vi "Center Front Panel.vi"(8 "error in (no error)":errorcluster, 11 "Actor in":refnum<class "Actor.lvclass">) -> (0 "error out":errorcluster, 3 "Actor out":refnum<class "Actor.lvclass">)   [LabVIEW 2015, in "Actor.lvclass"]
uses:
  Actor.lvclass
  Actor.lvclass/Actor.ctl
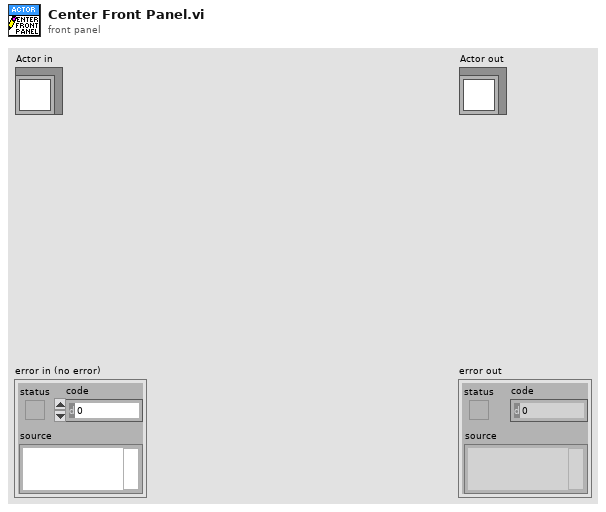
[diagram p1: front panel]
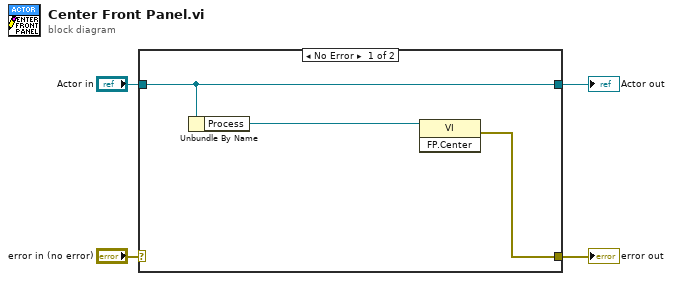
[diagram p0: block diagram]
diagram:
  n1 = case shown="No Error" "error in (no error)" {
    selector: "error in (no error)" -> [_ w8]
    tunnel: [w6 w8] -> w3
    tunnel: [w5 w9] -> w1
    tunnel: "Actor in" -> [w5 w9]
    frame No Error {
      n2 = Unbundle By Name(w5) -> ("Process"=w7:refnum<vi>)
      n3 = invoke class="VI" method="FP.Center"(reference=w7) -> (error out=w6:errorcluster)  [unwired: 2 in, 2 out]
    }
    frame Error {
    }
  }
  "error out" <- w3
  "Actor out" <- w1
